vi "vertcat.vi"(8 "error in (no error)":errorcluster, 9 "A1":dbl[][](array[numeric]), 10 "A0":dbl[][](array[numeric]), 11 "MatOper in":refnum<class "MatOper.lvclass">) -> (0 "error out":errorcluster, 2 "Stacked 2D Array":dbl[][](array[numeric]), 3 "MatOper out":refnum<class "MatOper.lvclass">)   [LabVIEW 2016, in "OfcFunc.lvlib" / "MatOper.lvclass"]
doc: "Vertical concatenate 2D arrays of A0 and A1. New 2D array is [A0, A1].T."
uses:
  MatOper.lvclass
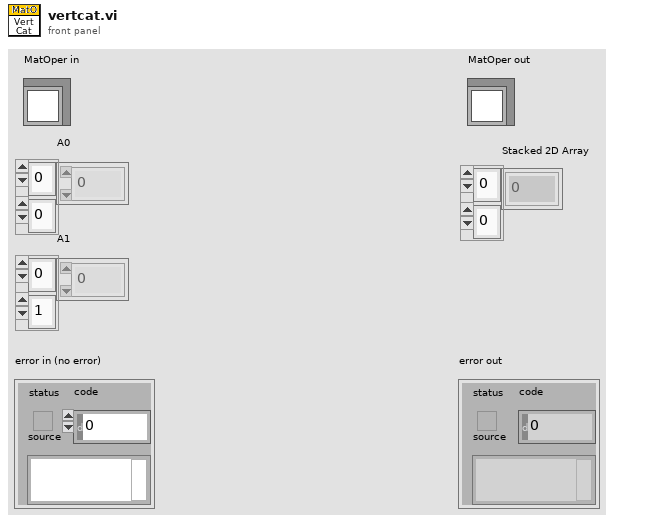
[diagram p1: front panel]
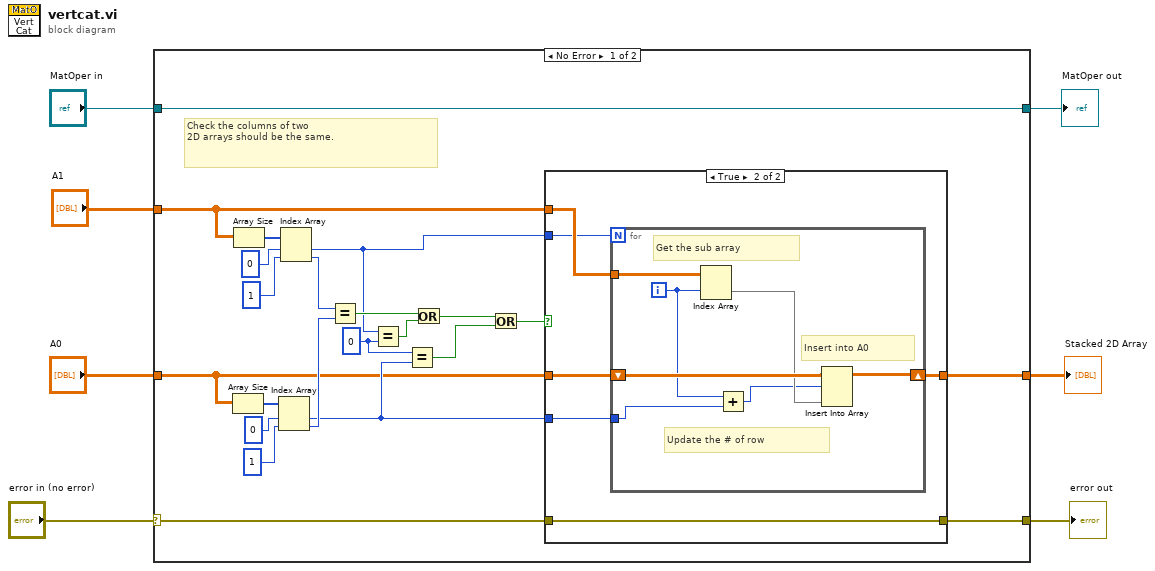
[diagram p0: block diagram]
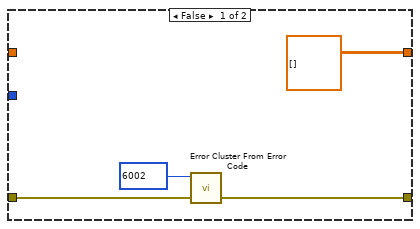
[diagram p2: hidden frame]
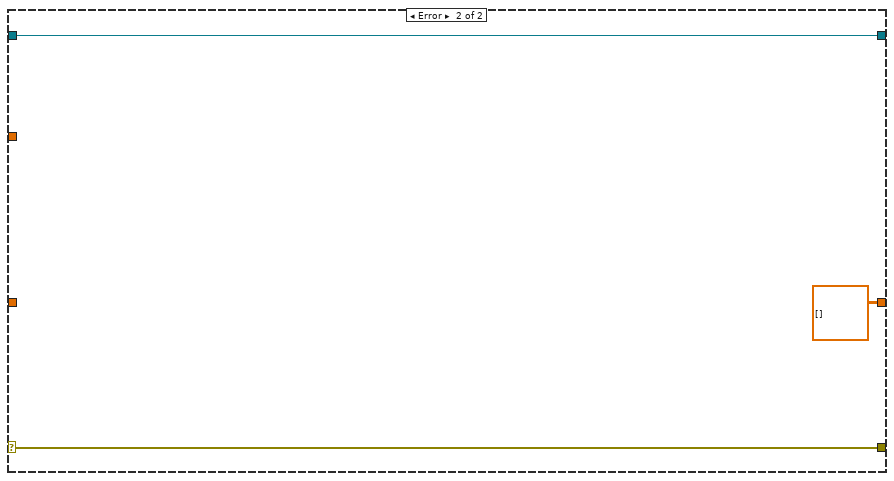
[diagram p3: hidden frame]
diagram:
  n1 = case shown="No Error" "error in (no error)" {
    selector: "error in (no error)" -> [w10 w49]
    tunnel: [w11 w49] -> w6
    tunnel: [w29 w48] -> w4
    tunnel: "MatOper in" -> [w29 w48]
    tunnel: [w12 dbl[][] [] ("A0")] -> w3
    tunnel: "A1" -> [w9 _]
    tunnel: "A0" -> [w8 _]
    frame No Error {
      w14 = 0 ("y")
      # "Check the columns of two\n2D arrays should be the same."
      n2 = Array Size(array=w8) -> (size(s)=w27:i32[])
      n3 = Array Size(array=w9) -> (size(s)=w28:i32[])
      n4 = Index Array(array=w27, index #1=0 ("index"), index #2=1 ("index")) -> (element #1=w13:i32, element #2=w21:i32)
      n5 = Index Array(array=w28, index #1=0 ("index"), index #2=1 ("index")) -> (element #1=w18:i32, element #2=w25:i32)
      n6 = Equal?(x=w25, y=w21) -> (x = y?=w20:bool)
      n7 = Equal?(x=w18, y=w14) -> (x = y?=w19:bool)
      n8 = Equal?(x=w14, y=w13) -> (x = y?=w16:bool)
      n9 = Or(x=w20, y=w19) -> (x .or. y?=w17:bool)
      n10 = Or(x=w17, y=w16) -> (x .or. y?=w15:bool)
      n11 = case shown="True" w15 {
        tunnel: [dbl[][] [] ("A0") w39] -> w12
        tunnel: w9 -> [_ w38]
        tunnel: w8 -> [_ w37]
        tunnel: w10 -> [w31 w36]
        tunnel: [w30 w36] -> w11
        tunnel: w18 -> [_ w35]
        tunnel: w13 -> [_ w34]
        frame False {
          n12 = call <vilib>:"Error Cluster From Error Code.vi"("error in (no error)"=w31, "error code (0)"=6002 ("code")) -> ("error out"=w30:errorcluster)  [unwired: 7 in]
        }
        frame True {
          n13 = for {
            N: w35 -> [_]
            shift-right: [w43] -> w39
            shift-left: w37 -> [w45]
            tunnel: w38 -> [w46]
            tunnel: w34 -> [w40]
            i -> [w41]
            # "Insert into A0"
            # "Get the sub array"
            # "Update the # of row"
            n14 = Index Array(array=w46, index (row)=w41) -> (element=w44:dbl[])  [unwired: 1 in]
            n15 = Add(x=w41, y=w40) -> (x+y=w42:i32)
            n16 = Insert Into Array(array=w45, index (row)=w42, new element=w44) -> (w43:dbl[][])  [unwired: 1 in]
          }
        }
      }
    }
    frame Error {
    }
  }
  "error out" <- w6
  "MatOper out" <- w4
  "Stacked 2D Array" <- w3
